vi "GetNumber.vi"(11 "COM Port":refnum<visa-resource-name>="COM3") -> (1 "String":string, 2 "Cluster":T1, 3 "VISA Output":refnum<visa-resource-name>)   [LabVIEW 2009]
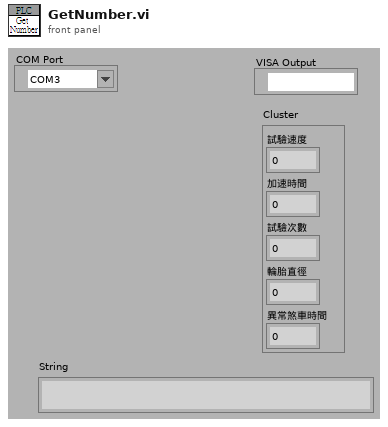
[diagram p1: front panel]
types:
  T1 = cluster{"試驗速度":u32, "加速時間":u32, "試驗次數":u32, "輪胎直徑":u32, "異常煞車時間":u32}
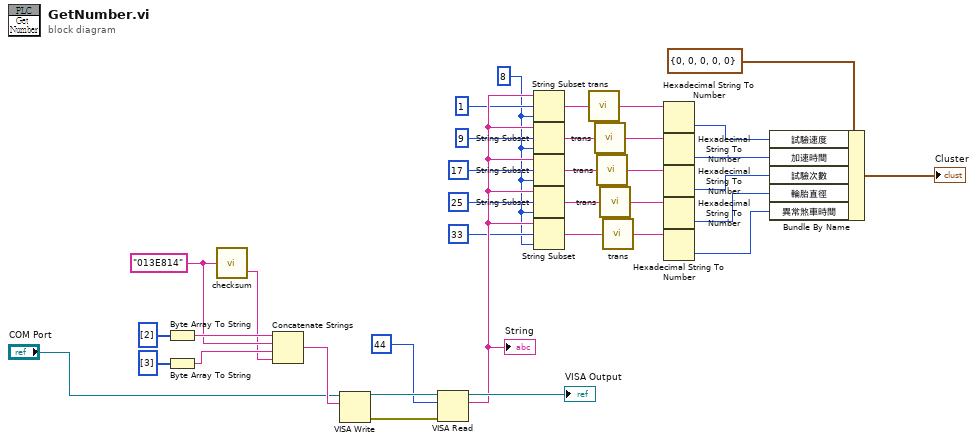
[diagram p0: block diagram]
diagram:
  w19 = 8
  w32 = "013E814"
  n1 = Byte Array To String(unsigned byte array=u8[] [2]) -> (string=w34:string)
  n2 = Byte Array To String(unsigned byte array=u8[] [3]) -> (string=w33:string)
  n3 = call "checksum.vi"("Data"=w32) -> ("Check Sum"=w31:string)  [unwired: 2 in, 1 out]
  n4 = Concatenate Strings(w34, w32, w33, w31) -> (w30:string)
  n5 = VISA Write(VISA resource name="COM Port", write buffer=w30) -> (VISA resource name out=w29:refnum<visa-resource-name>, error out=w28:errorcluster)  [unwired: 1 in, 1 out]
  n6 = VISA Read(VISA resource name=w29, byte count=u32 44, error in (no error)=w28) -> (VISA resource name out=→"VISA Output":refnum<visa-resource-name>, read buffer=w25:string)  [unwired: 2 out]
  "String" <- w25
  n7 = String Subset(string=w25, offset (0)=1, length (rest)=w19) -> (substring=w10:string)
  n8 = String Subset(string=w25, offset (0)=9, length (rest)=w19) -> (substring=w8:string)
  n9 = String Subset(string=w25, offset (0)=17, length (rest)=w19) -> (substring=w6:string)
  n10 = String Subset(string=w25, offset (0)=25, length (rest)=w19) -> (substring=w4:string)
  n11 = String Subset(string=w25, offset (0)=33, length (rest)=w19) -> (substring=w2:string)
  n12 = call "trans.vi"("String"=w10) -> ("String 2"=w9:string)
  n13 = call "trans.vi"("String"=w8) -> ("String 2"=w7:string)
  n14 = call "trans.vi"("String"=w6) -> ("String 2"=w5:string)
  n15 = call "trans.vi"("String"=w4) -> ("String 2"=w3:string)
  n16 = call "trans.vi"("String"=w2) -> ("String 2"=w1:string)
  n17 = Hexadecimal String To Number(string=w9) -> (number=w16:u32)  [unwired: 2 in, 1 out]
  n18 = Hexadecimal String To Number(string=w7) -> (number=w15:u32)  [unwired: 2 in, 1 out]
  n19 = Hexadecimal String To Number(string=w5) -> (number=w14:u32)  [unwired: 2 in, 1 out]
  n20 = Hexadecimal String To Number(string=w3) -> (number=w13:u32)  [unwired: 2 in, 1 out]
  n21 = Hexadecimal String To Number(string=w1) -> (number=w12:u32)  [unwired: 2 in, 1 out]
  n22 = Bundle By Name(cluster=T1 {"試驗速度"=0, "加速時間"=0, "試驗次數"=0, "輪胎直徑"=0, "異常煞車時間"=0} ("Cluster"), "試驗速度"=w16, "加速時間"=w15, "試驗次數"=w14, "輪胎直徑"=w13, "異常煞車時間"=w12) -> (→"Cluster":T1)
